vi "convU16[U8].vi"(1 "dimension size":i32=1 min=1 max=2 step=1, 2 "DATA IN":u16) -> (0 "DATA OUT":u8[](array[numeric]))   [LabVIEW 2023]
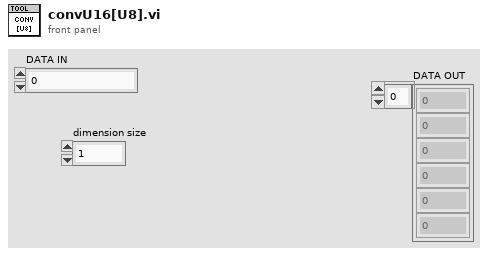
[diagram p1: front panel]
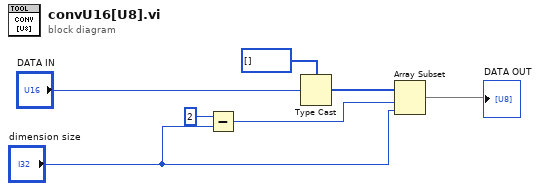
[diagram p0: block diagram]
diagram:
  n1 = Subtract(x=2, y="dimension size") -> (x-y=w2:i32)
  n2 = Type Cast(type=u8[] [], x="DATA IN") -> (*(type *) &x=w5:u8[])
  n3 = Array Subset(array=w5, index=w2, length="dimension size") -> (→"DATA OUT":u8[])
